vi "DownsampleStage2_5782.vi"(8 "valid in":bool, 9 "reset":bool, 11 "Data in":fxp<+/-,16,14>[](array[numeric])=[0.0, 0.0, 0.0, 0.0]) -> (0 "valid out":bool, 3 "data out":fxp<+/-,16,14>[](array[numeric]))   [LabVIEW 2013]
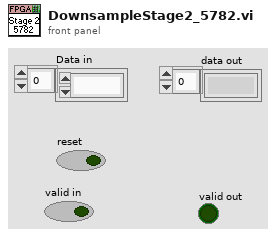
[diagram p1: front panel]
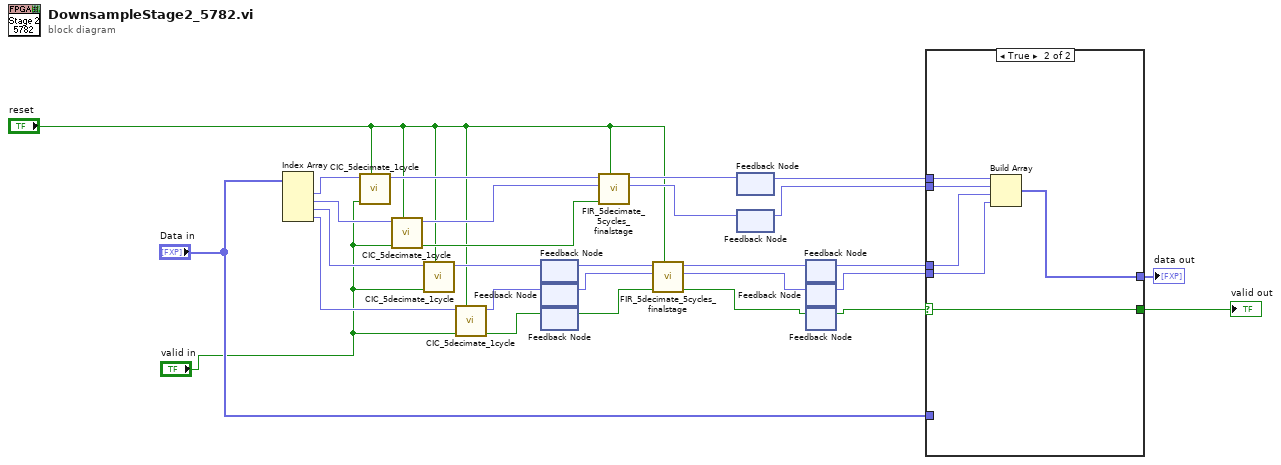
[diagram p0: block diagram]
diagram:
  n1 = Index Array(array="Data in") -> (element #1=w26:fxp<+/-,16,14>, element #2=w24:fxp<+/-,16,14>, element #3=w23:fxp<+/-,16,14>, element #4=w22:fxp<+/-,16,14>)  [unwired: 4 in]
  n2 = call "CIC_5decimate_1cycle.vi"("reset"="reset", "valid in"="valid in", "Data in"=w26) -> ("Data out"=w15:fxp<+/-,16,14>)  [unwired: 7 in, 1 out]
  n3 = call "CIC_5decimate_1cycle.vi"("reset"="reset", "valid in"="valid in", "Data in"=w24) -> ("valid out"=w13:bool, "Data out"=w14:fxp<+/-,16,14>)  [unwired: 7 in]
  n4 = call "CIC_5decimate_1cycle.vi"("reset"="reset", "valid in"="valid in", "Data in"=w23) -> ("Data out"=w21:fxp<+/-,16,14>)  [unwired: 7 in, 1 out]
  n5 = call "CIC_5decimate_1cycle.vi"("reset"="reset", "valid in"="valid in", "Data in"=w22) -> ("valid out"=w19:bool, "Data out"=w20:fxp<+/-,16,14>)  [unwired: 7 in]
  n6 = feedback #1() -> (w18:fxp<+/-,16,14>)  [unwired: 1 in]
  n7 = feedback-in #1(w21) -> ()
  n8 = feedback #2() -> (w17:fxp<+/-,16,14>)  [unwired: 1 in]
  n9 = feedback-in #2(w20) -> ()
  n10 = feedback #3() -> (w16:bool)  [unwired: 1 in]
  n11 = feedback-in #3(w19) -> ()
  n12 = call "FIR_5decimate_5cycles_finalstage.vi"("reset"="reset", "valid in"=w13, "Q in"=w14, "I in"=w15) -> ("Q out"=w11:fxp<+/-,16,14>, "I out"=w12:fxp<+/-,16,14>)  [unwired: 4 in, 2 out]
  n13 = call "FIR_5decimate_5cycles_finalstage.vi"("reset"="reset", "valid in"=w16, "Q in"=w17, "I in"=w18) -> ("valid out"=w4:bool, "Q out"=w5:fxp<+/-,16,14>, "I out"=w6:fxp<+/-,16,14>)  [unwired: 4 in, 1 out]
  n14 = feedback #4() -> (w10:fxp<+/-,16,14>)  [unwired: 1 in]
  n15 = feedback-in #4(w12) -> ()
  n16 = feedback #5() -> (w9:fxp<+/-,16,14>)  [unwired: 1 in]
  n17 = feedback-in #5(w11) -> ()
  n18 = feedback #6() -> (w2:fxp<+/-,16,14>)  [unwired: 1 in]
  n19 = feedback-in #6(w6) -> ()
  n20 = feedback #7() -> (w3:fxp<+/-,16,14>)  [unwired: 1 in]
  n21 = feedback-in #7(w5) -> ()
  n22 = feedback #8() -> (w1:bool)  [unwired: 1 in]
  n23 = feedback-in #8(w4) -> ()
  n24 = case shown="True" w1 {
    selector: w1 -> [w30 w36]
    tunnel: w10 -> [_ w35]
    tunnel: w9 -> [_ w34]
    tunnel: w2 -> [_ w32]
    tunnel: w3 -> [_ w33]
    tunnel: [w29 w31] -> w28
    tunnel: [w30 w36] -> w27
    tunnel: "Data in" -> [w29 _]
    frame False {
    }
    frame True {
      n25 = Build Array(w35, w34, w32, w33) -> (w31:fxp<+/-,16,14>[])
    }
  }
  "data out" <- w28
  "valid out" <- w27
